vi "clear_data_.vi"(6 "error in (no error)":errorcluster, 8 "dataIn":string) -> (0 "error out":errorcluster, 2 "dataOut":u32)   [LabVIEW 2021]
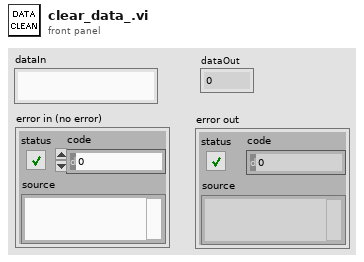
[diagram p1: front panel]
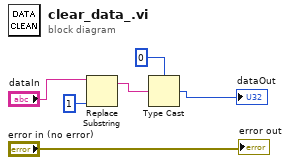
[diagram p0: block diagram]
diagram:
  n1 = Replace Substring(2:1 ("length (len. of substring)"), 5:"dataIn") -> (1:w1:string)  [unwired: 2 in, 1 out]
  n2 = Type Cast(type=u32 0, x=w1) -> (*(type *) &x=→"dataOut":u32)
  "error out" <- "error in (no error)"
